vi "Spectrometer Data.vi"(0 "VISA resource name":refnum<visa-resource-name>, 5 "Pixel Mode (0:Optical)":u16(ring) items=["Optical ", "All Pixels"], 7 "Ocean Optics Definitions":string[][](array[string])=[["name", "decimal number", "start black pixel", "stop black pixel", "start optical pixel", "stop optical", "All Pixels", "not usable", "note reference"], ["USB2000", "4098", "2", "24", "26", "2074", "3648", "0-1", ""], ["ADC1000", "4100", "0", "0", "26", "2047", "2048", "", ""], ["HR2000", "4106", "2", "24", "26", "2047", "2048", "0-1", "Note 1 "], ["HR4000", "4114", "6", "18", "22", "3669", "3648", "1-5 ,3670-3681", ""], ["HR2000+", "4118", "0", "17", "20", "2047", "2048", "18-19", ""], ["QE65000", "4120", "0 , 1038", "3 , 1043", "10", "1033", "1044", "4-9 , 1034-1037", "Note 2"], ["USB2000+", "4126", "2", "17", "20", "2047", "2048", "18-19", "Note 3"], ["USB4000", "4130", "6", "18", "22", "3669", "3648", "1-5,3670-3681", ""], ["NIRQuest512", "4134", "NaN", "", "0", "511", "1024", "", ""], ["NIRQuest256", "4136", "NaN", "", "0", "255", "512", "", ""], ["MAYA Pro", "4138", "1,2064", "3,067", "10", "2047", "2068", "0,4-9 ", ""], ["MAYA", "4140", "0,2072", "7,079", "16", "2063", "2080", "8,15-2064-2071", ""], ["Torus", "4160", "0", "17", "20", "2047", "2028", "18-19", ""], ["Flame", "4126", "2", "17", "20", "2047", "2048", "0", "0"]], 9 "Check Vrn First Call (False)":bool, 11 "error in (no error)":errorcluster) -> (2 "Name":string, 3 "Pixels":T1, 6 "USB Speed":u16, 8 "ID":u16, 10 "Optical Pixels":bool, 15 "error out":errorcluster)   [LabVIEW 2018, in "Ocean Optics 2000 4000.lvlib"]
doc: "Reads data (on first call) from the tables and uses it in subsequent calls.\n\nNote:\nIf changes are made to the data make sure to select Data Operations>> \"Make current values default\" before saving."
uses:
  Ocean Optics 2000 4000.lvlib
panel:
  in  "Notes":string[](array[string])=["Note:1 The HR2000 only digitizes the first 2048 pixels", "Note 2: In the QE6500 are the pixels 038..1047 (black pixels) in software moved to the back of the second set of black pixels.", "Note 3:  Per Ocean Optics tech support USB2000+ data sheet incorrectly labels 0-17 as dark pixels. Pixels 0 and 1 contain garbage and should not be used [AC]. The dark pixels are 2-17 [AC]. ", "Note 4: All Pixel values are from the Obsoleted Read Spectra VI"]
  # "The data is on first call read from the tables below and uses in subsequent calls\nIf you change the data make sure that you \"Make current values default\" before saving."
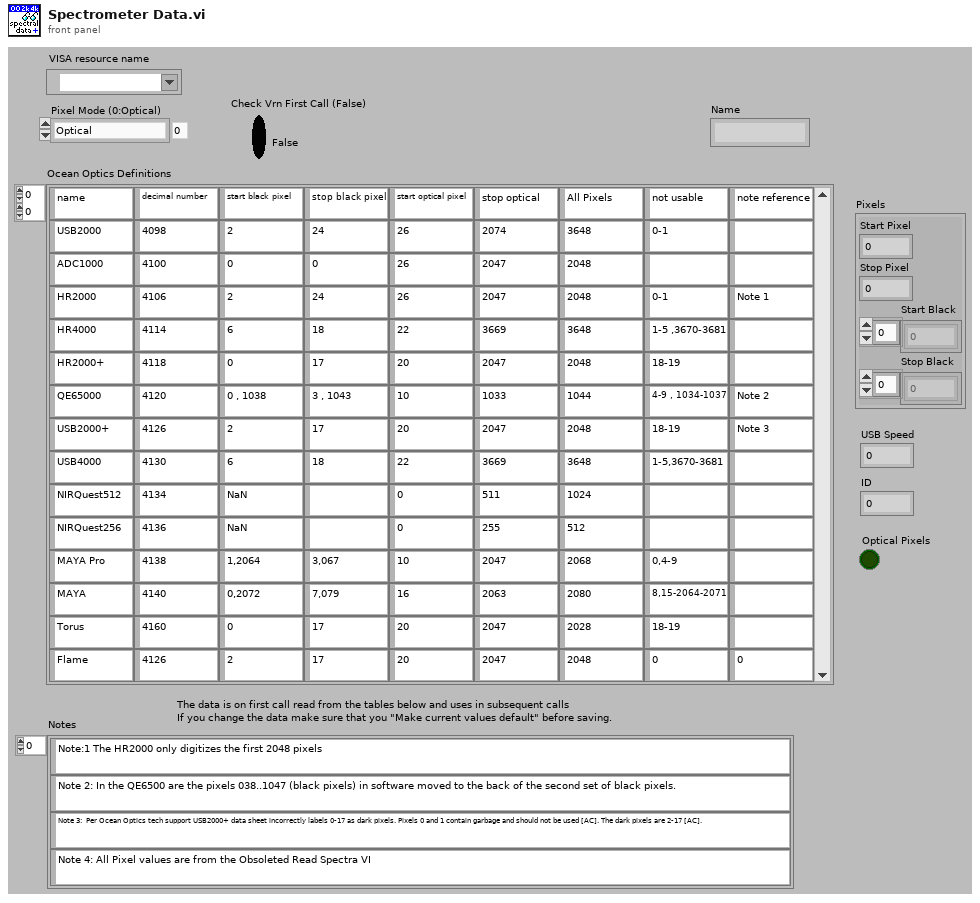
[diagram p1: front panel]
types:
  T1 = cluster{"Start Pixel":i32, "Stop Pixel":i32, "Start Black":i32[], "Stop Black":i32[]}
  T2 = cluster{"Start Pixel":i32, "Stop Pixel":i32, "Start Black":i32[], "Stop Black":i32[]}[]
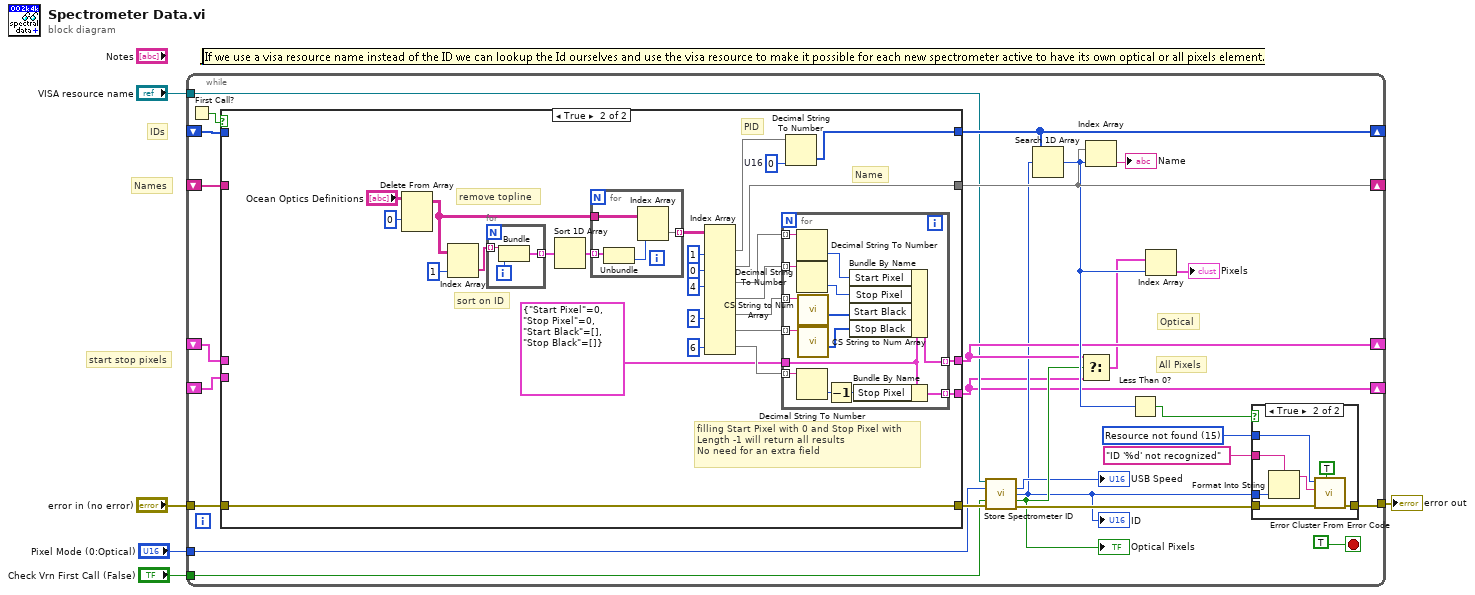
[diagram p0: block diagram]
diagram:
  # "start stop pixels"
  # "IDs"
  # "Names"
  n1 = while {
    shift-right: [w30] -> _
    shift-left: _ -> [w31]
    shift-right: [w28] -> _
    shift-left: _ -> [w29]
    shift-right: [w18] -> _
    shift-left: _ -> [w27]
    tunnel: [w24] -> w4
    tunnel: "error in (no error)" -> [w19]
    tunnel: "Pixel Mode (0:Optical)" -> [w12]
    shift-right: [w6] -> _
    shift-left: _ -> [w16]
    tunnel: "VISA resource name" -> [w11]
    tunnel: "Check Vrn First Call (False)" -> [w10]
    stop <- TRUE stop-if-true
    w21 = 15 items=["No error", "Argument error", "Memory is full", "Out of zone", "End of file", "File already open", "Generic file I/O error", "File not found", "File permission error", "Disk is full", "Duplicate path", "Too many files open", "System feature not enabled", "Resource file not found", "Cannot add resource", "Resource not found", "Image not found", "Image memory error", "Pen does not exist", "Config type invalid", "Config token not found", "Config parse error", "Config memory error", "Bad external code format", "Bad external code offset", "External code not present", "Null window", "Destroy window error", "Null menu", "Print aborted", "Bad print record", "Print driver error", "Windows error during printing", "Memory error during printing", "Print dialog error", "Generic print error", "Invalid device refnum", "Device not found", "Device parameter error", "Device unit error", "Cannot open device", "Device call aborted", "Generic error", "Cancelled by user", "Object ID too low", "Object ID too high", "Object not in heap", "Unknown heap", "Unknown object (invalid DefProc)", "Unknown object (DefProc not in table)", "Message out of range", "Invalid (null) method", "Unknown message", "Manager call not supported", "Bad address", "Network operation in progress", "Network operation timed out", "Connection is busy", "Network attribute not supported", "Network error", "Address in use", "System out of memory", "Connection aborted", "Connection refused", "Not connected", "Already connected", "Connection closed", "Initialization error (interapplication manager)", "Bad occurrence", "Wait on unbound occurrence handler", "Occurrence queue overflow", "Datalog type conflict", "Unused", "Unrecognized type (interapplication manager)", "Memory corrupt", "Failed to make temporary DLL", "Old CIN version", "Drag socket not found", "Failed to load drop-object", "Failed to register OLE object", "Failed to release OLE object", "Format specifier type mismatch", "Unknown format specifier", "Too few format specifiers", "Too many format specifiers", "Scan failed", "Newer CIN version", "Error converting to variant", "Runtime menu error", "Password tampered", "Variant attribute not found", "Incompatible variant data type", "Event data is not available", "Event Store is not present", "Occurrence is not found", "Event Queue is not created", "Event info is not available", "Refnum passed is NULL", "Error retrieving Class GUID", "Error retrieving CoClass GUID", "Error retrieving TypeLib GUID.", "Bad built application magic bytes.", "Specific driver is different from the specific driver associated with the Logical Name.", "There is no session opened to the class driver.", "Max Error", "MAX - Error with config objects", "MAX - Error loading configuration", "MAX - Group not supported"] ("error code enum (Argument error)")
    # "All Pixels"
    # "Optical"
    n2 = First Call?() -> (First Call?: T/F=w32:bool)
    n3 = case shown="True" w32 {
      tunnel: [w44 w54] -> w28
      tunnel: w31 -> [w45 _]
      tunnel: [w45 w51] -> w30
      tunnel: w29 -> [w44 _]
      tunnel: [w43 w56] -> w18
      tunnel: w27 -> [w43 _]
      tunnel: w19 -> [w42 w50]
      tunnel: [w42 w50] -> w14
      tunnel: [w41 w47] -> w6
      tunnel: w16 -> [w41 _]
      frame False {
      }
      frame True {
        w55 = u16 0  # U16
        # "filling Start Pixel with 0 and Stop Pixel with\nLength -1 will return all results\nNo need for an extra field"
        # "PID"
        # "Name"
        # "remove topline"
        # "sort on ID"
        n4 = Delete From Array(array="Ocean Optics Definitions", index (row)=0) -> (array with subset deleted=w65:string[][])  [unwired: 2 in, 1 out]
        n5 = Index Array(array=w65, index (col)=1 ("disabled index (col)")) -> (element=w71:string[])  [unwired: 1 in]
        n6 = for {
          tunnel: w71 -> [w90] mode=indexing
          tunnel: [w92] -> w69 mode=indexing
          i -> [w91]
          n7 = Bundle("String"=w90, w91) -> (w92:cluster{"String":string, i32})  [unwired: 1 out]
        }
        n8 = Sort 1D Array(array=w69) -> (sorted array=w68:cluster{"String":string, i32}[])
        n9 = for {
          tunnel: w68 -> [w86] mode=indexing
          tunnel: w65 -> [w89]
          tunnel: [w87] -> w64 mode=indexing
          n10 = Unbundle(w86) -> (w88:i32)  [unwired: 1 out]
          n11 = Index Array(array=w89, index (row)=w88) -> (element=w87:string[])  [unwired: 1 in]
        }
        n12 = Index Array(array=w64, index (col) #1=1 ("disabled index (col)"), index (col) #2=0 ("index (col)"), index (col) #3=4 ("index (col)"), index (col) #5=2 ("index (col)"), index (col) #7=6 ("index (col)")) -> (element #1=w52:string[], element #2=w51:string[], element #3=w62:string[], element #4=w61:string[], element #5=w59:string[], element #6=w57:string[], element #7=w48:string[])  [unwired: 9 in]
        n13 = for {
          tunnel: w62 -> [w85] mode=indexing
          tunnel: w61 -> [w84] mode=indexing
          tunnel: w59 -> [w74] mode=indexing
          tunnel: w57 -> [w76] mode=indexing
          tunnel: T1 {"Start Pixel"=0, "Stop Pixel"=0, "Start Black"=[], "Stop Black"=[]} ("Pixels") -> [w78]
          tunnel: [w81] -> w56 mode=indexing
          tunnel: w48 -> [w80] mode=indexing
          tunnel: [w77] -> w47 mode=indexing
          n14 = Decimal String To Number(string=w85) -> (number=w83:i32)  [unwired: 2 in, 1 out]
          n15 = Decimal String To Number(string=w84) -> (number=w82:i32)  [unwired: 2 in, 1 out]
          n16 = Decimal String To Number(string=w80) -> (number=w79:i32)  [unwired: 2 in, 1 out]
          n17 = call "CS String to Num Array.vi"("String"=w74) -> ("Positions"=w73:i32[])  [unwired: 10 in]
          n18 = call "CS String to Num Array.vi"("String"=w76) -> ("Positions"=w75:i32[])  [unwired: 10 in]
          n19 = Decrement(x=w79) -> (x-1=w72:i32)
          n20 = Bundle By Name(cluster=w78, "Start Pixel"=w83, "Stop Pixel"=w82, "Start Black"=w73, "Stop Black"=w75) -> (w81:T1)
          n21 = Bundle By Name(cluster=w78, "Stop Pixel"=w72) -> (w77:T1)
        }
        n22 = Decimal String To Number(string=w52, default (0L)=w55) -> (number=w54:u16[])  [unwired: 1 in, 1 out]
      }
    }
    n23 = call "Store Spectrometer ID.vi"("VISA resource name"=w11, "Pixel Mode (0:Optical)"=w12, "Check Vrn First Call (False)"=w10, "error in (no error)"=w14) -> ("USB Speed"=→"USB Speed":u16, "ID"=w7:u16, "Optical Pixels"=w9:bool, "error out"=w13:errorcluster)  [unwired: 7 in, 1 out]
    "Optical Pixels" <- w9
    "ID" <- w7
    n24 = Search 1D Array(1D array=w28, element=w7) -> (index of element=w23:i32)  [unwired: 1 in]
    n25 = Select(t=w18, s=w9, f=w6) -> (s? t:f=w17:T2)
    n26 = Index Array(array=w30, index=w23) -> (element=→"Name":string)
    n27 = Less Than 0?(x=w23) -> (x < 0?=w22:bool)
    n28 = Index Array(array=w17, index=w23) -> (element=→"Pixels":T1)
    n29 = case shown="True" w22 {
      tunnel: w13 -> [w33 w39]
      tunnel: [w33 w38] -> w24
      tunnel: w7 -> [_ w36]
      tunnel: w21 -> [_ w37]
      tunnel: "ID '%d' not recognized" -> [_ w35]
      frame False {
      }
      frame True {
        n30 = Format Into String(format string=w35, w36) -> (resulting string=w34:string)  [unwired: 2 in, 1 out]
        n31 = call <vilib>:"Error Cluster From Error Code.vi"("show call chain? (False)"=TRUE, "error in (no error)"=w39, "error message (\"\")"=w34, "error code (0)"=w37) -> ("error out"=w38:errorcluster)  [unwired: 5 in]
      }
    }
  }
  "error out" <- w4
